vi "Get Laser Drive.vi"(8 "error in (no error)":errorcluster, 9 "Path":path, 10 "Section":string, 11 "Test Station SIM LASER Factory in":refnum<class "Test Station SIM LASER Factory.lvclass">) -> (0 "error out":errorcluster, 2 "Laser Driver.lvclass":refnum<class "Laser Driver.lvclass">)   [LabVIEW 2022 SP3, in "Test Station SIM LASER Factory.lvclass"]
uses:
  Test Station SIM LASER Factory.lvclass
  Test Station SIM LASER Factory.lvclass/Test Station SIM LASER Factory.ctl
  Sim Laser Driver/Sim Laser Driver.lvclass
  Test Station SIM Laser Driver/Test Station SIM Laser Driver.lvclass
  C:/XY Stage/Laser/Sim Laser Driver/Sim Laser Driver.lvclass
  C:/XY Stage/XY Stage/Framework/Base/Base.lvclass
  C:/XY Stage/Laser/Laser Driver/Laser Driver.lvclass
  C:/XY Stage/Laser/Test Station SIM Laser Driver/Test Station SIM Laser Driver.lvclass
  Test Station SIM Laser Driver/Action.ctl
  Laser Driver/Laser Driver.lvclass
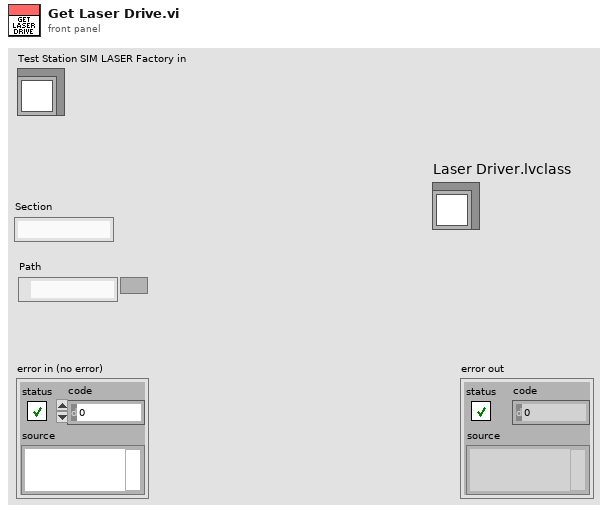
[diagram p1: front panel]
types:
  T1 = typedef "Test Station SIM Laser Driver.lvclass/Action.ctl" = enum16{"Read Data", "Set Data"}
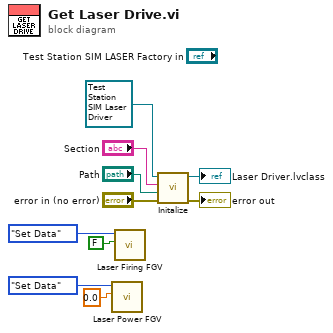
[diagram p0: block diagram]
diagram:
  n1 = call "Laser Power FGV.vi"("Laser Power"=0.0, "Action"=Action."Set Data") -> ()  [unwired: 8 in, 2 out]
  n2 = call "Laser Firing FGV.vi"("Laser Firing"=FALSE, "Action"=Action."Set Data") -> ()  [unwired: 8 in, 2 out]
  n3 = call "Initalize.vi"("error in (no error)"="error in (no error)", "Path"="Path", "Section"="Section", "Sim Laser Driver in"=refnum<class "Test Station SIM Laser Driver.lvclass"> refnum ("Test Station SIM Laser Driver.lvclass")) -> ("error out"=→"error out":errorcluster, "Sim Laser Driver out"=→"Laser Driver.lvclass":refnum<class "Test Station SIM Laser Driver.lvclass">)  [unwired: 6 in]
